vi "CAD@AddPart(FromPartModel)__Parameter.vi"(1 "ParamterIn":string) -> (0 "ParamterOut":string)   [LabVIEW 2020]
panel:
  in  "PartName":string(combo)
  in  "PartModel":string(combo)
  in  "Confirm":bool
  # "CAD@AddPart(FromPartModel) $PartModel,$ParName1(,$PartName2....)"
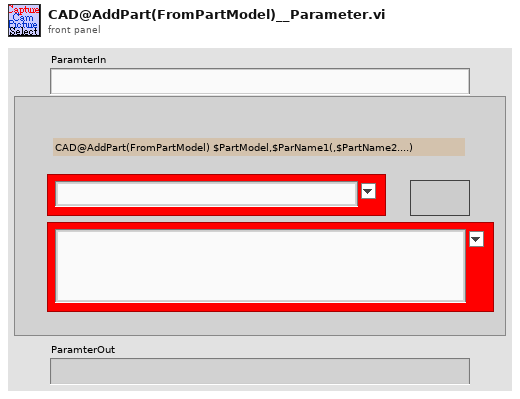
[diagram p1: front panel]
types:
  T1 = enum16{"Init", "Load Tool", "Load Part", "Get Tool Property", "Get Part Property", "Set Tool to End Matrix", "Set Part to Tool Matrix", "Calculate Part to Tool & End Matrix", "Create Part From Copy", "Delete Part"}
  T2 = cluster{"Tool Name":string[], "Part Name":string[]}
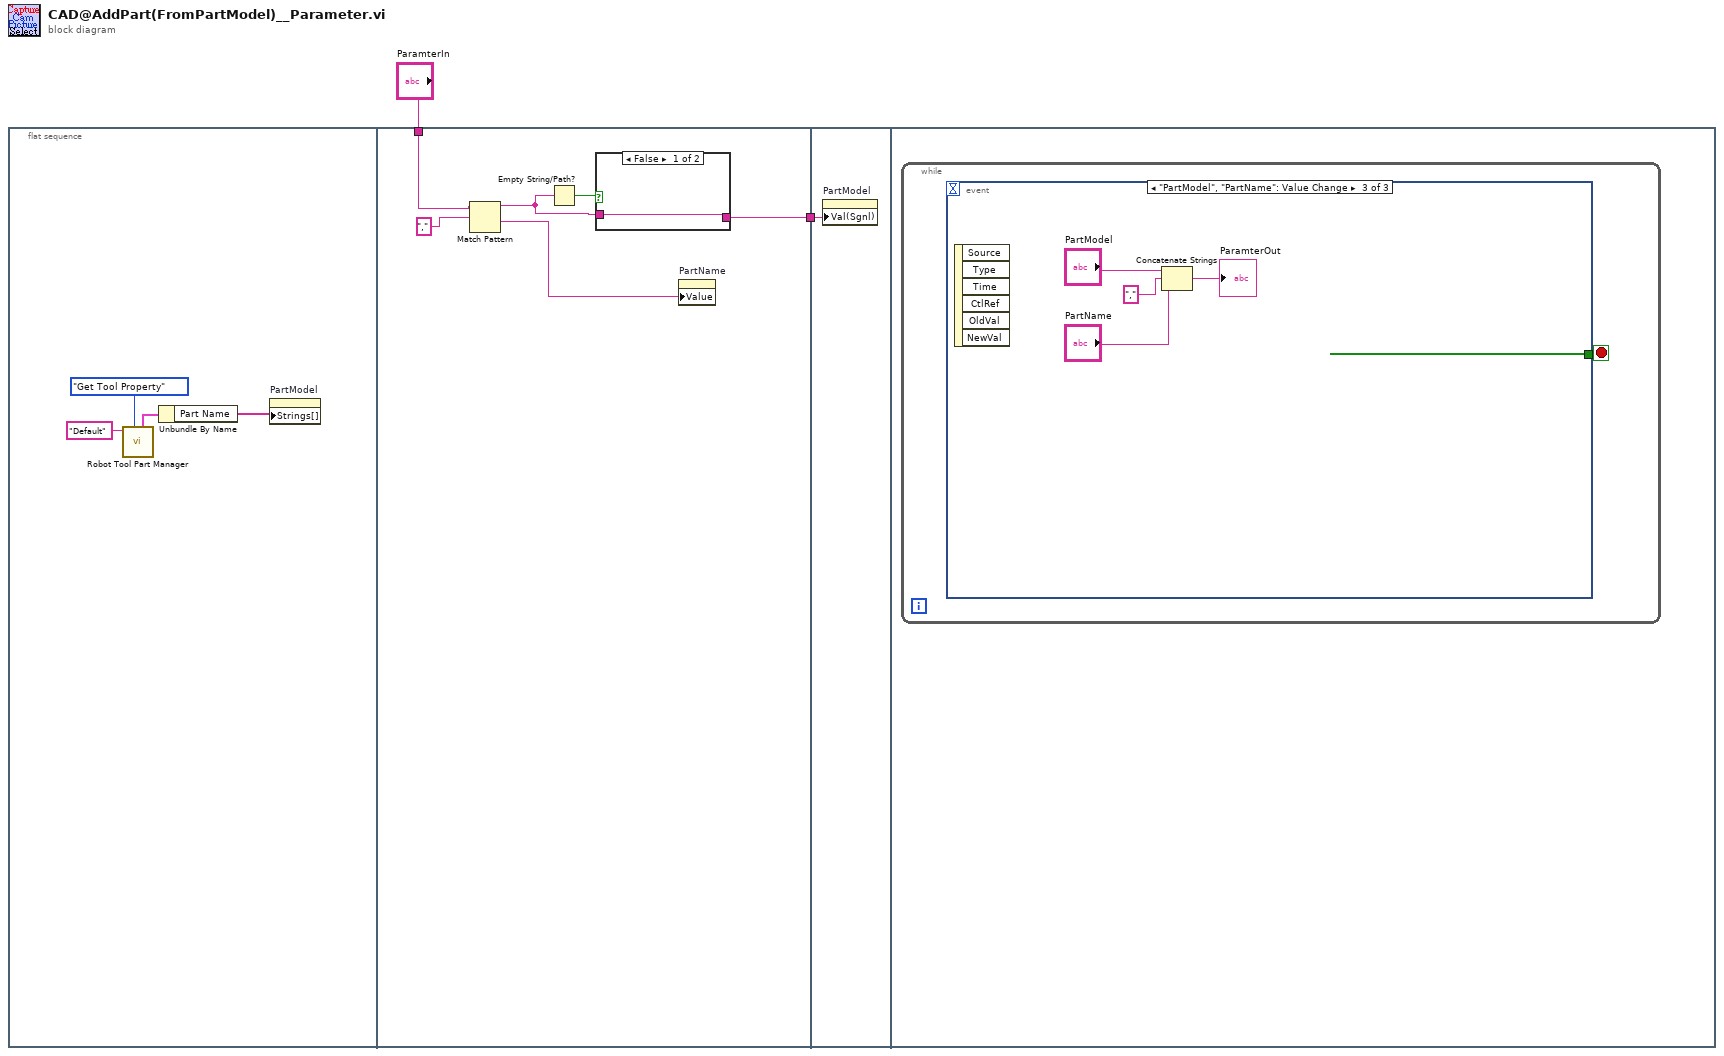
[diagram p0: block diagram]
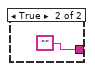
[diagram p2: hidden frame]
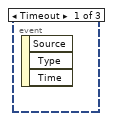
[diagram p3: hidden frame]
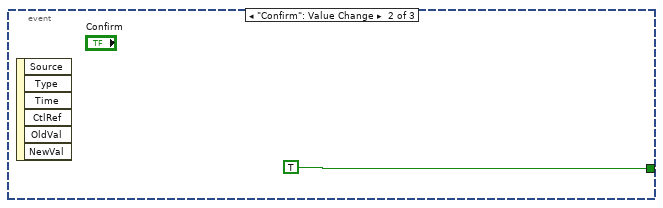
[diagram p4: hidden frame]
diagram:
  n1 = flat-sequence {
    tunnel: "ParamterIn" -> [w10]
    tunnel: [w11] -> w1
    tunnel: w1 -> [w15]
    frame #0 {
      n2 = call "Robot Tool Part Manager.vi"("CMD"=T1."Get Tool Property", "Tool / Part Name"="Default") -> ("NameList"=w4:T2)  [unwired: 4 in, 5 out]
      n3 = Unbundle By Name(w4) -> ("Part Name"=w3:string[])
      n4 = property on="PartModel" class="CmbBox"("Strings[]"=w3) -> ()  [unwired: 2 in, 2 out]
    }
    frame #1 {
      n5 = Match Pattern(string=w10, regular expression="," ("search string/char (-)")) -> (before substring=w8:string, after substring=w7:string)  [unwired: 1 in, 2 out]
      n6 = Empty String/Path?(string/path=w8) -> (empty?=w12:bool)
      n7 = case shown="False" w12 {
        tunnel: [w13 ""] -> w11
        tunnel: w8 -> [w13 _]
        frame False {
        }
        frame True {
        }
      }
      n8 = property on="PartName" class="CmbBox"("Value"=w7) -> ()  [unwired: 2 in, 2 out]
    }
    frame #2 {
      n9 = property on="PartModel" class="CmbBox"("Val(Sgnl)"=w15) -> ()  [unwired: 2 in, 2 out]
    }
    frame #3 {
      n10 = while {
        stop <- w16 stop-if-true
        n11 = event shown="[2] \"PartModel\", \"PartName\": Value Change" {
          selector: _ -> [_ _ _]
          dyn-events: _ -> [_ _ _]
          timeout: _ -> [_ _ _]
          tunnel: [_ TRUE _] -> w16
          event Timeout {
            n12 = event-data() -> ()  [unwired: 1 in, 3 out]
          }
          event "Confirm": Value Change {
            n13 = event-data() -> ()  [unwired: 1 in, 6 out]
          }
          event "PartModel", "PartName": Value Change {
            n14 = event-data() -> ()  [unwired: 1 in, 6 out]
            n15 = Concatenate Strings("PartModel", ",", "PartName") -> (→"ParamterOut":string)
          }
        }
      }
    }
  }
